vi "s_CloseMotor.vi"(1 "Error In":errorcluster, 2 "Motor Reference In":refnum<k7>) -> (0 "Error Out":errorcluster)   [LabVIEW 2014]
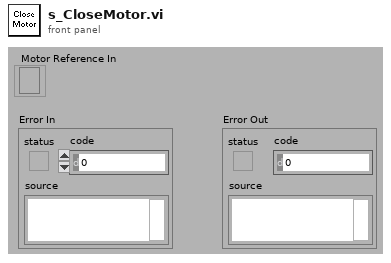
[diagram p1: front panel]
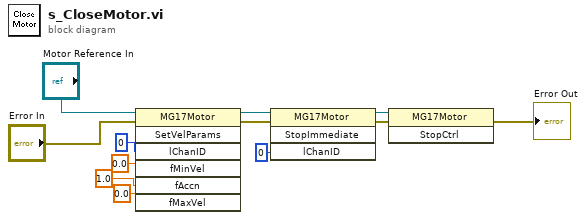
[diagram p0: block diagram]
diagram:
  n1 = invoke class="MG17Motor" method="SetVelParams"(reference="Motor Reference In", error in="Error In", "lChanID"=0, "fMinVel"=sgl 0.0, "fAccn"=sgl 1.0, "fMaxVel"=sgl 0.0) -> (reference out=w6:refnum<k7>, error out=w7:errorcluster)  [unwired: 1 in, 5 out]
  n2 = invoke class="MG17Motor" method="StopImmediate"(reference=w6, error in=w7, "lChanID"=0) -> (reference out=w8:refnum<k7>, error out=w9:errorcluster)  [unwired: 1 in, 2 out]
  n3 = invoke class="MG17Motor" method="StopCtrl"(reference=w8, error in=w9) -> (error out=→"Error Out":errorcluster)  [unwired: 1 in, 2 out]
